vi "Find All Direction.vi"(5 "Primary Direction":T1, 7 "Present(f) Not Present(t)":bool, 10 "Target Array":i32[](array[numeric]), 11 "View":i32[](array[numeric])) -> (2 "Direction Array Out":T1[](array[typedef]), 3 "Found":bool)   [LabVIEW 2016, in "AntFarm_MB.lvclass"]
uses:
  AntFarm_MB.lvclass
  Type Defs/Direction Enum.ctl
  Type Defs/SB Type Defs.lvlib
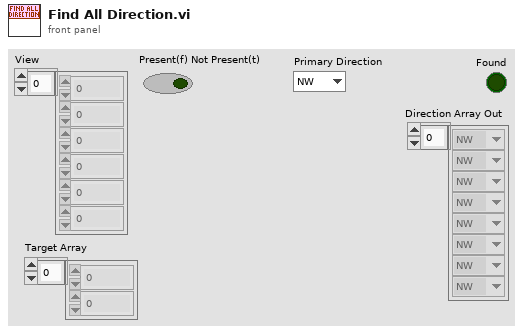
[diagram p1: front panel]
types:
  T1 = typedef "SB Type Defs.lvlib/Direction Enum.ctl" = enum16{"NW", "N", "NE", "E", "SE", "S", "SW", "W"}
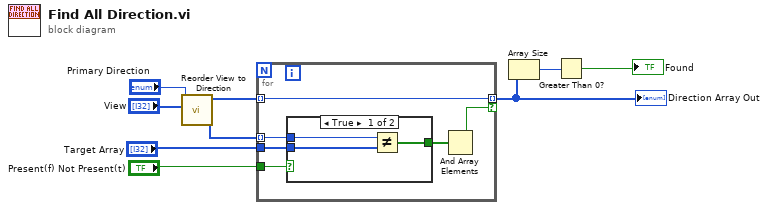
[diagram p0: block diagram]
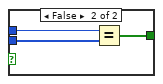
[diagram p2: hidden frame]
diagram:
  n1 = call "Reorder View to Direction.vi"("View in"="View", "Primary Direction"="Primary Direction") -> ("View out"=w1:i32[], "Direction List"=w3:T1[])  [unwired: 8 in]
  n2 = for {
    tunnel: w1 -> [w13] mode=indexing
    tunnel: "Target Array" -> [w15]
    tunnel: [w10] -> w7 mode=indexing if=w11
    tunnel: "Present(f) Not Present(t)" -> [w12]
    tunnel: w3 -> [w10] mode=indexing
    n3 = case shown="True" w12 {
      tunnel: w15 -> [w18 w21]
      tunnel: [w17 w20] -> w14
      tunnel: w13 -> [w16 w19]
      frame True {
        n4 = Not Equal?(x=w16, y=w18) -> (x != y?=w17:bool[])
      }
      frame False {
        n5 = Equal?(x=w19, y=w21) -> (x = y?=w20:bool[])
      }
    }
    n6 = And Array Elements(Boolean array=w14) -> (logical AND=w11:bool)
  }
  "Direction Array Out" <- w7
  n7 = Array Size(array=w7) -> (size(s)=w6:i32)
  n8 = Greater Than 0?(x=w6) -> (x > 0?=→"Found":bool)
